vi "Create Pipe.vi"(8 "error in (no error)":errorcluster, 10 "permissions (664)":T1={"owner"={"read"=TRUE, "write"=TRUE, "execute"=FALSE}, "group"={"read"=TRUE, "write"=TRUE, "execute"=FALSE}, "everyone"={"read"=TRUE, "write"=FALSE, "execute"=FALSE}}, 11 "pathname in":string) -> (0 "error out":errorcluster, 2 "pipe already exists?":bool, 3 "pathname out":string)   [LabVIEW 2013, in "Linux RT IPC.lvlib" / "Pipes.lvlib"]
doc: "This VI creates a new pipe in the filesystem at the path provided. The created pipe can be opened by writer and reader endpoints to transfer data."
uses:
  Pipes.lvlib
  C/C.lvlib
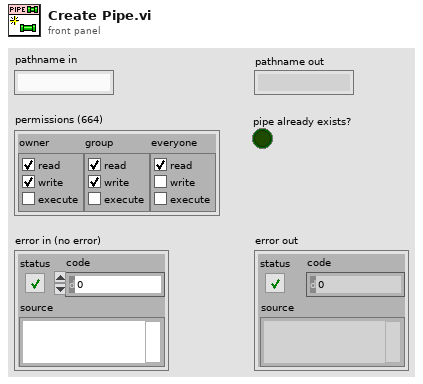
[diagram p1: front panel]
types:
  T1 = cluster{"owner":cluster{"read":bool, "write":bool, "execute":bool}, "group":cluster{"read":bool, "write":bool, "execute":bool}, "everyone":cluster{"read":bool, "write":bool, "execute":bool}}
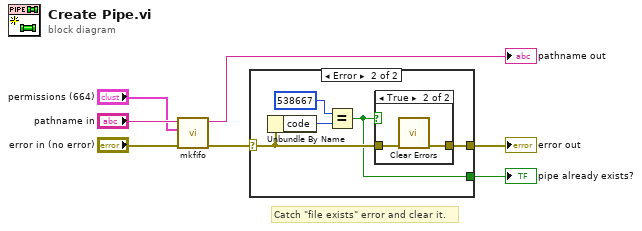
[diagram p0: block diagram]
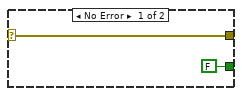
[diagram p2: hidden frame]
diagram:
  # "Catch \"file exists\" error and clear it."
  n1 = call "mkfifo.vi"("error in (no error)"="error in (no error)", "permissions (664)"="permissions (664)", "pathname in"="pathname in") -> ("error out"=w3:errorcluster, "pathname out"=→"pathname out":string)  [unwired: 7 in]
  n2 = case shown="Error" w3 {
    selector: w3 -> [w9 w12]
    tunnel: [w9 w13] -> w2
    tunnel: [FALSE w10] -> w1
    frame No Error {
    }
    frame Error {
      n3 = Unbundle By Name(w12) -> ("code"=w14:i32)
      n4 = Equal?(x=538667, y=w14) -> (x = y?=w10:bool)
      n5 = case shown="True" w10 {
        tunnel: w12 -> [w15 w17]
        tunnel: [w15 w16] -> w13
        frame False {
        }
        frame True {
          n6 = call <vilib>:"Clear Errors.vi"("error in (no error)"=w17) -> ("error out"=w16:errorcluster)  [unwired: 6 in]
        }
      }
    }
  }
  "error out" <- w2
  "pipe already exists?" <- w1
